vi "get_AgentID.vi"(8 "error in (no error)":errorcluster, 11 "MoAgSy_Engine.lvclass in":refnum<class "MoAgSy_Engine.lvclass">) -> (0 "error out":errorcluster, 1 "destination":string, 2 "Agent ID":string, 3 "MoAgSy_Engine.lvclass out":refnum<class "MoAgSy_Engine.lvclass">)   [LabVIEW 2009, in "MoAgSy.lvlib" / "MoAgSy_Engine.lvclass"]
uses:
  MoAgSy_Engine.lvclass
  MoAgSy_Engine.lvclass/MoAgSy_Engine.ctl
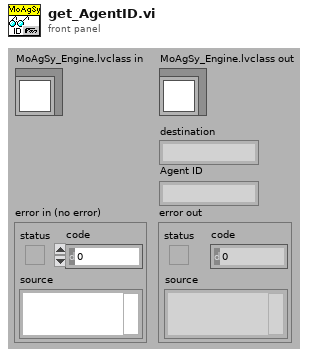
[diagram p1: front panel]
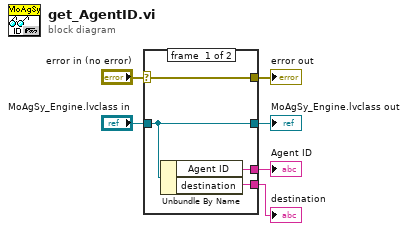
[diagram p0: block diagram]
diagram:
  n1 = case shown="No Error" "error in (no error)" {
    selector: "error in (no error)" -> [w10 w11]
    tunnel: [w10 w11] -> w5
    tunnel: [w9 w12] -> w3
    tunnel: "MoAgSy_Engine.lvclass in" -> [w9 w12]
    tunnel: [w8 _] -> w2
    tunnel: [w7 _] -> w1
    frame #0 {
      n2 = Unbundle By Name(w9) -> ("Agent ID"=w8:string, "destination"=w7:string)
    }
    frame #1 {
    }
  }
  "error out" <- w5
  "MoAgSy_Engine.lvclass out" <- w3
  "Agent ID" <- w2
  "destination" <- w1
